vi "(RIGHT)alignment by encoders for rotation.vi"(5 "On/Off":bool=TRUE, 8 "error in (no error)":errorcluster) -> (0 "error out":errorcluster)   [LabVIEW 2017]
uses:
  <vilib>/myRIO/Common/Instrument Driver Framework/myRIO v1.0/Encoder/typedefs/Encoder Signal Mode.ctl
  <vilib>/myRIO/Instrument Drivers/Onboard IO/Encoder/typedefs/Encoder Reference.ctl
  <vilib>/myRIO/Common/Instrument Driver Framework/Utilities/typedefs/myRIO Generic Hardware Reference.ctl
  <vilib>/myRIO/Common/Instrument Driver Framework/Utilities/typedefs/Hardware Version Enum.ctl
  <vilib>/myRIO/Common/Instrument Driver Framework/Utilities/typedefs/myRIO v1.0 Reference.ctl
  <vilib>/myRIO/Common/Instrument Driver Framework/Utilities/typedefs/Generic FPGA Reference.ctl
  <vilib>/myRIO/Common/Instrument Driver Framework/myRIO v1.0/Encoder/typedefs/Encoder Channels Enum.ctl
  <vilib>/myRIO/Common/Instrument Driver Framework/myRIO v1.0/Encoder/typedefs/Encoder Configuration v1.0.ctl
  <vilib>/userdefined/High Color/nirio_resource_hc.ctl
  <vilib>/myRIO/Common/Instrument Driver Framework/Utilities/vis/Is FPGA Ref Available.vi
  <vilib>/myRIO/Common/Instrument Driver Framework/myRIO v1.0/Encoder/vis/myRIO v1.1 Open Encoder.vi
  <vilib>/myRIO/Instrument Drivers/Onboard IO/Encoder/vis/Read.vi
  <vilib>/myRIO/Common/Instrument Driver Framework/Utilities/vis/Validate Channels.vi
  <vilib>/myRIO/Common/Instrument Driver Framework/myRIO v1.0/Encoder/vis/myRIO v1.0 Reserve Encoder.vi
  <vilib>/myRIO/Common/Instrument Driver Framework/myRIO v1.0/Encoder/vis/myRIO v1.0 Build MUX Configuration Encoder.vi
  <vilib>/myRIO/Common/Instrument Driver Framework/myRIO v1.0/Resource Manager/vis/myRIO v1.0 Reserve Channel List.vi
  <vilib>/myRIO/Common/Instrument Driver Framework/myRIO v1.0/Resource Manager/vis/myRIO v1.0 Create Configuration List.vi
  <vilib>/myRIO/Common/Instrument Driver Framework/myRIO v1.0/Resource Manager/vis/myRIO v1.0 Reserve Channel.vi
  <vilib>/myRIO/Common/Instrument Driver Framework/myRIO v1.0/Resource Manager/vis/myRIO v1.0 Unreserve Channel.vi
  <vilib>/myRIO/Common/Instrument Driver Framework/myRIO v1.0/Resource Manager/vis/myRIO v1.0 Build Mutex Name.vi
  <vilib>/Utility/VariantDataType/GetNumericInfo.vi
  <vilib>/Utility/error.llb/Error Cluster From Error Code.vi
  <vilib>/myRIO/Common/Instrument Driver Framework/myRIO v1.0/myRIO v1.1 Open.vi
  <vilib>/myRIO/Common/Instrument Driver Framework/Utilities/vis/IO Manager.vi
  <vilib>/myRIO/Common/Instrument Driver Framework/Utilities/vis/Configuration Manager.vi
  <vilib>/myRIO/Common/Instrument Driver Framework/myRIO v1.0/Resource Manager/vis/myRIO v1.0 Configure IO.vi
  <vilib>/myRIO/Common/Instrument Driver Framework/myRIO v1.0/myRIO v1.0 Close.vi
  <vilib>/myRIO/Common/Instrument Driver Framework/myRIO v1.0/Encoder/vis/myRIO v1.0 Configure Encoder.vi
  <vilib>/myRIO/Common/Instrument Driver Framework/myRIO v1.0/Encoder/vis/myRIO v1.0 Read Encoder.vi
  <vilib>/imath/engines/lvmath2/RunTimeEngine/Managers/WorkSpace/UID Generator.vi
  <vilib>/imath/engines/lvmath2/RunTimeEngine/RunTimeType/NIMS_RunTimeType_From StrictType (excl LVString).vi
  <instcachedir>/0/NIMS_RunTimeType_From StrictType (excl LVString)_1019F277F0A747EDBCA0F6C52CA54500.lvgen/NIMS_RunTimeType_From StrictType (excl LVString)_1019F277F0A747EDBCA0F6C52CA54500_000.vi
  <vilib>/imath/engines/lvmath2/RunTimeEngine/LocalVariableDefStatement/MC_LocalVariableDefStatement_Display.vi
  <vilib>/imath/engines/lvmath2/RunTimeEngine/RunTimeType/NIMS_RunTimeType_Set Source Original Bool.vi
  <vilib>/imath/engines/lvmath2/RunTimeEngine/VariableToken/NIMS_VariableToken_CondDefined.vi
  <instcachedir>/0/NIMS_VariableToken_CondDefined_6E7F1EE7F80E48298C84CF05BD736261.lvgen/NIMS_VariableToken_CondDefined_6E7F1EE7F80E48298C84CF05BD736261_004.vi
  <vilib>/imathl/engines/lvmath/Functions/Error Handling/Create Error.vi
  <vilib>/imath/engines/lvmath/Functions/Error Handling/MergeErrorsWrapper.vi
  <vilib>/imath/engines/lvmath2/RunTimeEngine/Managers/SymbolTable/Clear UID.vi
  <vilib>/imath/engines/lvmath2/RunTimeEngine/NodeEndStatement/NIMS_NodeEndStatement_Output.vi
  <instcachedir>/0/NIMS_NodeEndStatement_Output_53EC0D466D134D7ABD903AC30B43404B.lvgen/NIMS_NodeEndStatement_Output_53EC0D466D134D7ABD903AC30B43404B_010.vi
  <instcachedir>/0/NIMS_NodeEndStatement_Output_53EC0D466D134D7ABD903AC30B43404B.lvgen/NIMS_NodeEndStatement_Output_53EC0D466D134D7ABD903AC30B43404B_013.vi
  <vilib>/imath/engines/lvmath2/RunTimeEngine/ErrorHandling/NIMS_Finalize Error.vi
  <vilib>/myRIO/Express VI/Onboard IO/Encoder/Encoder Express VI.xnode
  <vilib>/myRIO/Instrument Drivers/Onboard IO/Encoder/vis/myRIO Encoder Open.xnode
  <vilib>/myRIO/Common/Instrument Driver Framework/myRIO v1.0/Encoder/typedefs/Encoder Count Direction Enum.ctl
  <vilib>/myRIO/Instrument Drivers/Onboard IO/Encoder/Encoder.lvlib
  <vilib>/imath/engines/lvmath2/RunTimeEngine/Managers/SymbolTable/NIMS_WorkSpace.lvlib
panel:
  in  "Reset Counter":bool
  out "Enc_left":ext
  out "current":ext
  in  "left":bool
  in  "right":bool
  out "right 2":bool
  out "left 2":bool
  out "Enc_right":ext
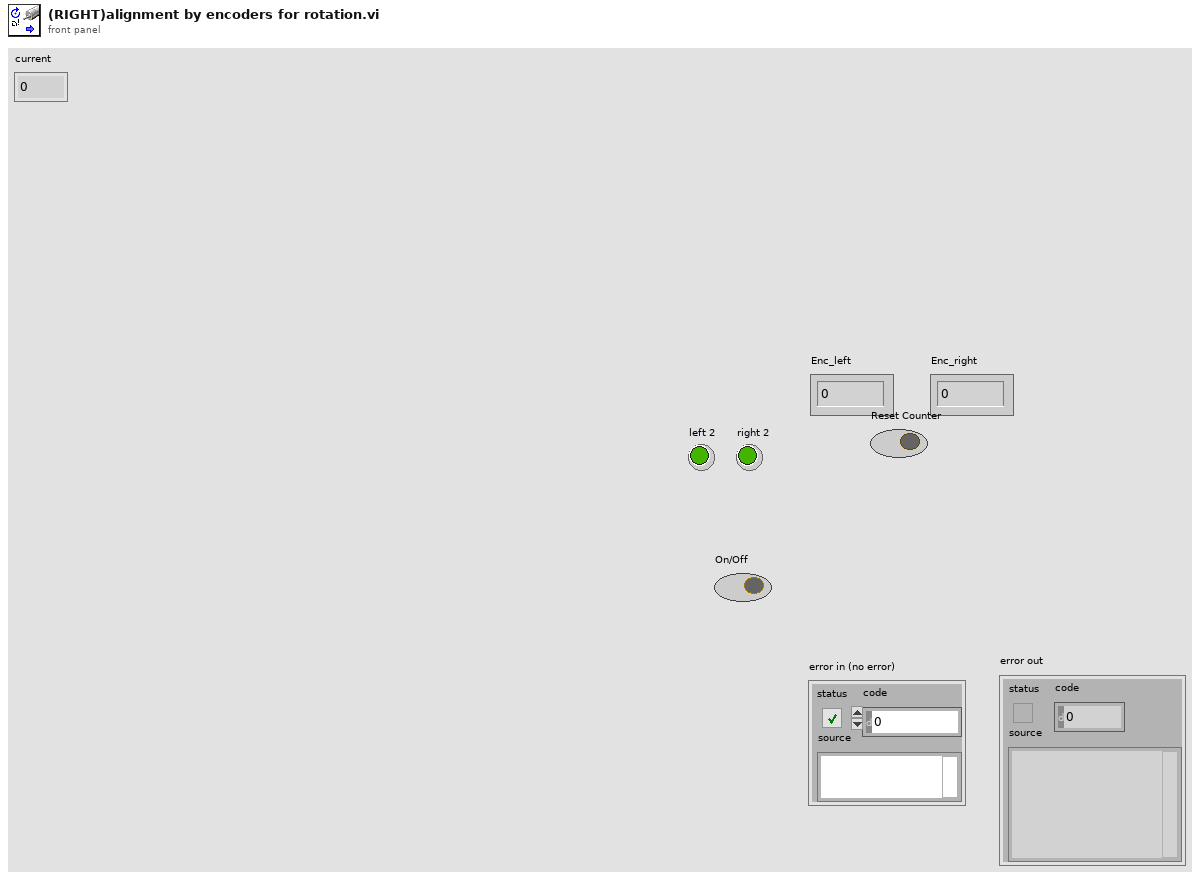
[diagram p1: front panel]
types:
  T1 = typedef "Encoder.lvlib/Encoder Reference.ctl" = cluster{"myRIO Reference":T2, "Encoder Channels Enum":T6}
  T2 = typedef "myRIO Generic Hardware Reference.ctl" = cluster{"myRIO Model":T3, "myRIO Hardware Reference":T4}
  T3 = typedef "Hardware Version Enum.ctl" = enum16{"Unknown", "myRIO-1900", "myRIO-1950", "roboRIO", "NI ELVIS RIO CM"}
  T4 = typedef "myRIO v1.0 Reference.ctl" = cluster{"Generic FPGA Reference":T5, "Allow multiple opens":bool}
  T5 = typedef "Generic FPGA Reference.ctl" = refnum<k20>
  T6 = typedef "Encoder Channels Enum.ctl" = enum16{"Not Connected", "C/ENC0", "C/ENC1", "A/ENC", "B/ENC", "DIO/ENC0", "DIO/ENC1", "DIO/ENC2", "DIO/ENC3", "DIO/ENC4"}
  T7 = typedef "Encoder Signal Mode.ctl" = enum16{"Quadrature phase signal", "Step and direction signal"}
  T8 = typedef "nirio_resource_hc.ctl" = tag
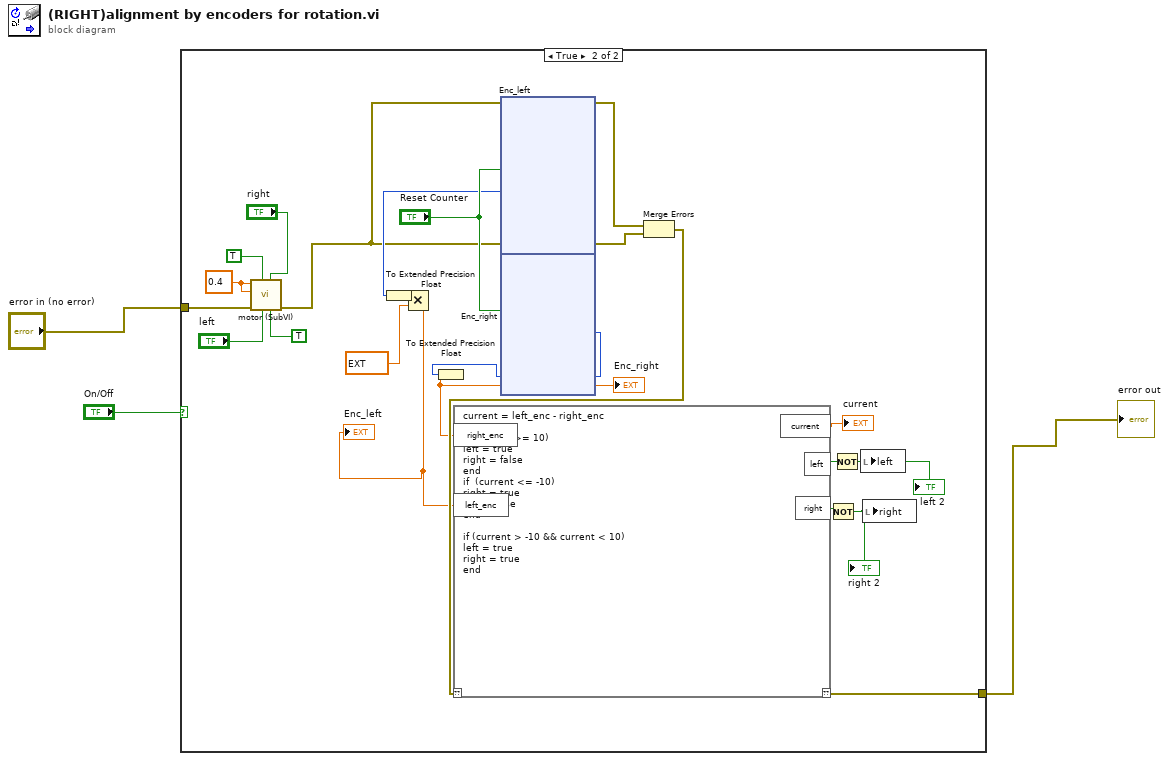
[diagram p0: block diagram]
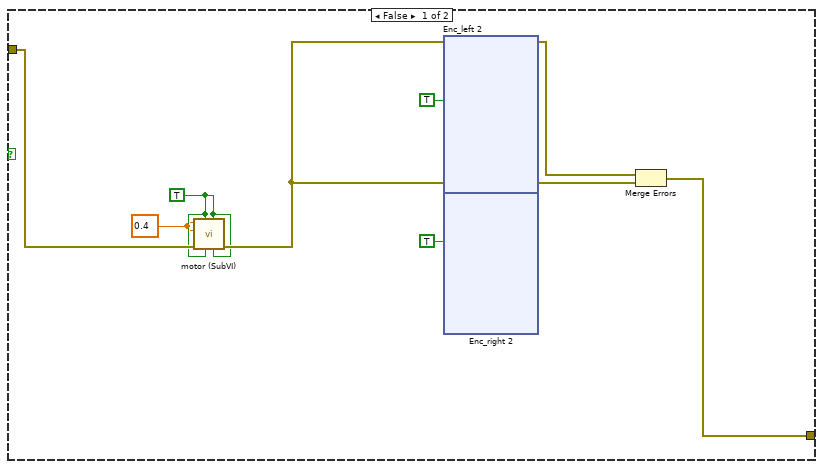
[diagram p2: hidden frame]
diagram:
  n1 = case shown="True" "On/Off" {
    tunnel: "error in (no error)" -> [w9 w127]
    tunnel: [w8 w126] -> w2
    frame False {
      w4 = 0.4 ("PWM1")
      w5 = TRUE ("M0 (Pin 21)")
      n2 = call "motor (SubVI).vi"("M1 (Pin 26)"=w5, "M1 (Pin 25)"=w5, "M0 (Pin 23)"=w5, "M0 (Pin 21)"=w5, "error in (no error)"=w9, "PWM1"=w4, "PWM0"=w4) -> ("error out"=w12:errorcluster)  [unwired: 4 in]
      n3 = xnode "Enc_left 2"("Reset Counter"=TRUE, "error in (no error)"=w12) -> ("error out"=w7:errorcluster)  [unwired: 3 out]
      n4 = xnode "Enc_right 2"("Reset Counter"=TRUE, "error in (no error)"=w12) -> ("error out"=w6:errorcluster)  [unwired: 3 out]
      n5 = Merge Errors(w7, w6) -> (w8:errorcluster)
    }
    frame True {
      w112 = 0.4 ("PWM0")
      n6 = call "motor (SubVI).vi"("M1 (Pin 26)"=TRUE, "M1 (Pin 25)"="right", "M0 (Pin 23)"="left", "M0 (Pin 21)"=TRUE, "error in (no error)"=w127, "PWM1"=w112, "PWM0"=w112) -> ("error out"=w111:errorcluster)  [unwired: 4 in]
      n7 = xnode "Enc_left"("Reset Counter"="Reset Counter", "error in (no error)"=w111) -> ("Counter Value"=w120:i32, "error out"=w125:errorcluster)  [unwired: 2 out]
      n8 = To Extended Precision Float(1:w120) -> (0:w114:ext)
      n9 = Multiply(x=w114, y=ext 0.865) -> (x*y=w113:ext)
      "Enc_left" <- w113
      n10 = xnode "Enc_right"("Reset Counter"="Reset Counter", "error in (no error)"=w111) -> ("Counter Value"=w119:i32, "error out"=w124:errorcluster)  [unwired: 2 out]
      n11 = To Extended Precision Float(1:w119) -> (0:w115:ext)
      "Enc_right" <- w115
      n12 = Merge Errors(w125, w124) -> (w121:errorcluster)
      n13 = mathscript code="current = left_enc - right_enc\n\nif (current >= 10)\nleft = true\nright = false\nend\nif  (current <= -10)\nright = true\nleft = false\nend\n\nif (current > -10 && current < 10)\nleft = true\nright = true\nend"("??"=w121, "left_enc"=w113, "right_enc"=w115) -> ("??"=w126:errorcluster, "current"=→"current":ext, "left"=w117:bool, "right"=w118:bool)
      n14 = Not(x=w118) -> (.not. x?=w109:bool)
      "right 2" <- w109
      n15 = Not(x=w117) -> (.not. x?=w110:bool)
      "left 2" <- w110
      n16 = local write "left"(w110) -> ()
      n17 = local write "right"(w109) -> ()
    }
  }
  "error out" <- w2
